vi "Mech Calculate_Drive_Power_Nemo_Style.vi"(6 "Power":sgl=100.0, 7 "Reverse":bool, 8 "Deadband (10)":i8=10 min=0 max=100 step=1, 10 "Controller State":T1={"Left X"=0, "Left Y"=0, "Right X"=0, "Right Y"=0, "Button Encoding 9-12"=0, "Button Encoding 1-8"=0, "POV"=-1} {"POV" items=["None"=-1, "POV Up"=0, "POV Up Right"=1, "POV Right"=2, "POV Down Right"=3, "POV Down"=4, "POV Down Left"=5, "POV Left"=6, "POV Up Left"=7]}) -> (0 "Right Rear Power":i8, 1 "Right Front Power":i8, 2 "Left Rear Power":i8, 3 "Left Front Power":i8)   [LabVIEW 2012]
doc: "Determines the amount of power to apply to a set of motors according to the x and y values of two joysticks on a game controller for a mecanum drive train.\n\n<B>Inputs</B>\n<B>Power Level</B> specifies the maximum amount of power to apply to the motor. For example, a value of 50 scales the fuznge of the joystick to a range of -50 to 50. A negative value drives the motor with the same power as its equivalent positive number but in the opposite direction. You can specify a value between -100 and 100. A value of 0 specifies the motor does not move. The default is 50.\n<B>Controller State</B> specifies the values of the joystick axes and button states of the game controller.\n<B>Deadband</B> specifies the joystick values that the VI treats as zero. When the position of the joystick is within the range you specify, the VI considers the joystick to be at position 0. The default range is -10 to 10.\n\n<B>Outputs</B>\n<B>Left Front Motor Power</B> returns the amount of power to apply to the left front motor. \n<B>Left Rear Motor Power</B> returns the amount of power to apply to the left rear motor. \n<B>Right Front Motor Power</B> returns the amount of power to apply to the right front motor.\n<B>Right Rear Motor Power</B> returns the amount of power to apply to the right rear motor.\n\nLF power = Ly + Rx + Lx\nRF power = Ly - Rx - Lx\nLR power = Ly + Rx - Lx\nRR power = Ly - Rx +Lx"
uses:
  <vilib>/FTC/FTC ControllerState.ctl
  <vilib>/FTC/FTC POVState.ctl
  <vilib>/NXT/Dual Mode Library/prims/inRangeAndCoerce/inRangeAndCoerce_float.vi
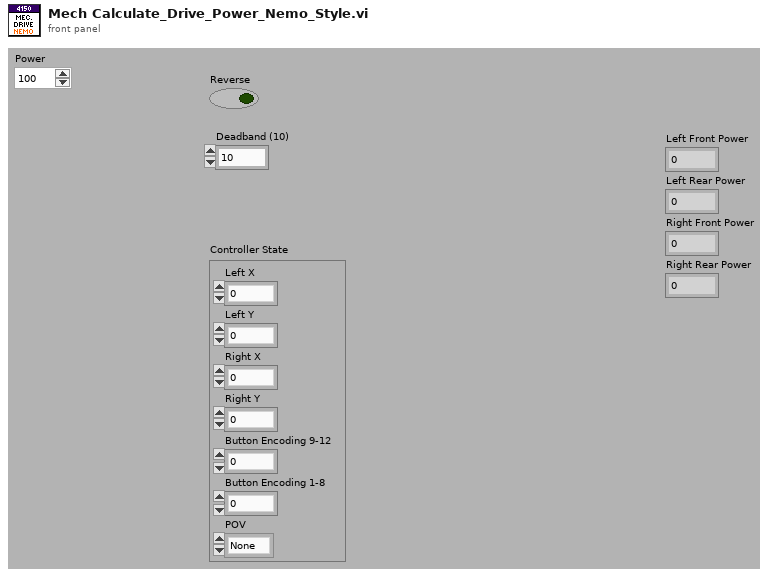
[diagram p1: front panel]
types:
  T1 = typedef "FTC ControllerState.ctl" = cluster{"Left X":i8, "Left Y":i8, "Right X":i8, "Right Y":i8, "Button Encoding 9-12":u8, "Button Encoding 1-8":u8, "POV":T2}
  T2 = typedef "FTC POVState.ctl" = i8
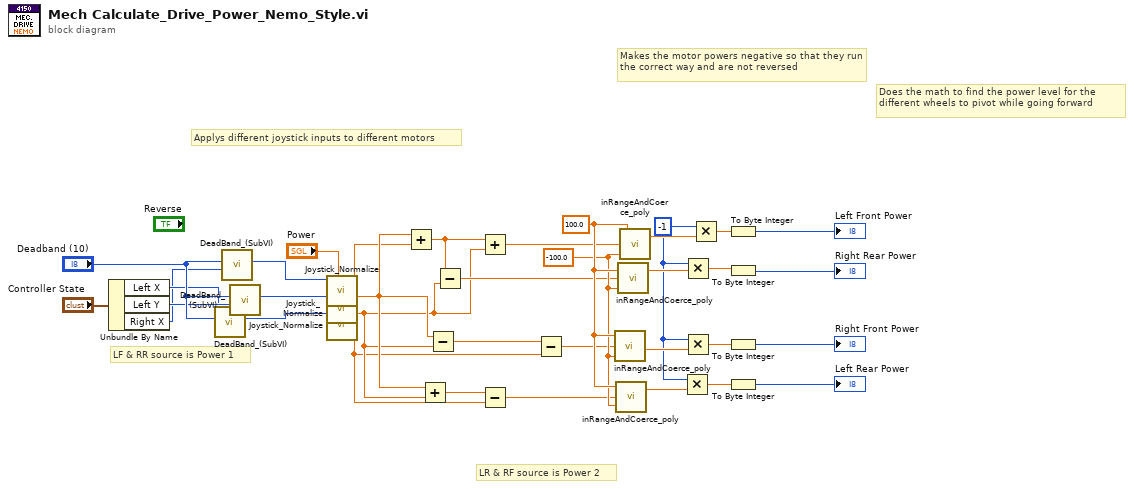
[diagram p0: block diagram]
diagram:
  w4 = -1
  w30 = sgl -100.0 ("lower limit")
  w31 = sgl 100.0 ("upper limit")
  # "Makes the motor powers negative so that they run the correct way and are not reversed"
  # "Does the math to find the power level for the \ndifferent wheels to pivot while going forward"
  # "Applys different joystick inputs to different motors"
  # "LR & RF source is Power 2"
  # "LF & RR source is Power 1"
  n1 = Unbundle By Name("Controller State") -> ("Left X"=w2:i8, "Left Y"=w32:i8, "Right X"=w1:i8)
  n2 = call "DeadBand_(SubVI).vi"("Axis In"=w2, "Deadband (10)"="Deadband (10)") -> ("Axis out"=w28:i8)  [unwired: 9 in]
  n3 = call "DeadBand_(SubVI).vi"("Axis In"=w1, "Deadband (10)"="Deadband (10)") -> ("Axis out"=w27:i8)  [unwired: 9 in]
  n4 = call "DeadBand_(SubVI).vi"("Axis In"=w32, "Deadband (10)"="Deadband (10)") -> ("Axis out"=w29:i8)  [unwired: 9 in]
  n5 = call "Joystick_Normalize.vi"("Power"="Power", "Joystick In"=w27) -> ("Norm Out"=w3:sgl)  [unwired: 9 in]
  n6 = call "Joystick_Normalize.vi"("Power"="Power", "Joystick In"=w29) -> ("Norm Out"=w16:sgl)  [unwired: 9 in]
  n7 = call "Joystick_Normalize.vi"("Power"="Power", "Joystick In"=w28) -> ("Norm Out"=w15:sgl)  [unwired: 9 in]
  n8 = Add(x=w16, y=w3) -> (x+y=w20:sgl)
  n9 = Add(x=w16, y=w15) -> (x+y=w14:sgl)
  n10 = Subtract(x=w16, y=w15) -> (x-y=w18:sgl)
  n11 = Subtract(x=w20, y=w15) -> (x-y=w19:sgl)
  n12 = Add(x=w20, y=w15) -> (x+y=w21:sgl)
  n13 = Subtract(x=w14, y=w3) -> (x-y=w13:sgl)
  n14 = Subtract(x=w18, y=w3) -> (x-y=w17:sgl)
  n15 = call-poly <vilib>:"inRangeAndCoerce_poly.vi"("lower limit"=w30, "x"=w17, "upper limit"=w31) -> ("coerced(x)"=w6:sgl)  [unwired: 1 out]
  n16 = call-poly <vilib>:"inRangeAndCoerce_poly.vi"("lower limit"=w30, "x"=w13, "upper limit"=w31) -> ("coerced(x)"=w5:sgl)  [unwired: 1 out]
  n17 = call-poly <vilib>:"inRangeAndCoerce_poly.vi"("lower limit"=w30, "x"=w19, "upper limit"=w31) -> ("coerced(x)"=w8:sgl)  [unwired: 1 out]
  n18 = call-poly <vilib>:"inRangeAndCoerce_poly.vi"("lower limit"=w30, "x"=w21, "upper limit"=w31) -> ("coerced(x)"=w11:sgl)  [unwired: 1 out]
  n19 = Multiply(x=w4, y=w5) -> (x*y=w9:sgl)
  n20 = Multiply(x=w4, y=w8) -> (x*y=w7:sgl)
  n21 = Multiply(x=w4, y=w6) -> (x*y=w10:sgl)
  n22 = Multiply(x=w4, y=w11) -> (x*y=w12:sgl)
  n23 = To Byte Integer(number=w12) -> (8bit integer=→"Left Front Power":i8)
  n24 = To Byte Integer(number=w7) -> (8bit integer=→"Right Rear Power":i8)
  n25 = To Byte Integer(number=w10) -> (8bit integer=→"Right Front Power":i8)
  n26 = To Byte Integer(number=w9) -> (8bit integer=→"Left Rear Power":i8)
